vi "Remove Spurious.vi"(5 "Min V":dbl, 6 "Init":bool, 7 "Min I":dbl, 9 "VOLTS":dbl, 11 "Current":dbl) -> (0 "V Out":dbl, 3 "I Out":dbl)   [LabVIEW 2017]
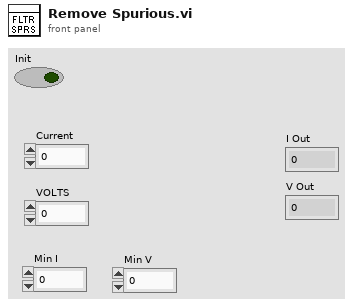
[diagram p1: front panel]
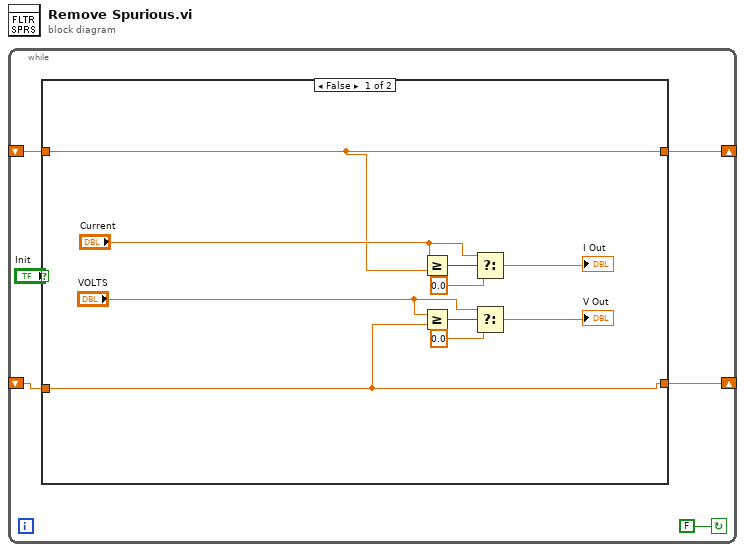
[diagram p0: block diagram]
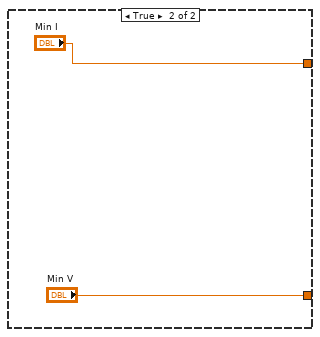
[diagram p2: hidden frame]
diagram:
  n1 = while {
    shift-right: [w3] -> _
    shift-left: _ -> [w2]
    shift-right: [w4] -> _
    shift-left: _ -> [w1]
    stop <- FALSE continue-if-true
    n2 = case shown="False" "Init" {
      tunnel: [w7 "Min V"] -> w4
      tunnel: [w8 "Min I"] -> w3
      tunnel: w2 -> [w8 _]
      tunnel: w1 -> [w7 _]
      frame False {
        n3 = Greater Or Equal?(x="Current", y=w8) -> (x >= y?=w11:bool)
        n4 = Greater Or Equal?(x="VOLTS", y=w7) -> (x >= y?=w15:bool)
        n5 = Select(t="Current", s=w11, f=0.0) -> (s? t:f=→"I Out":dbl)
        n6 = Select(t="VOLTS", s=w15, f=0.0) -> (s? t:f=→"V Out":dbl)
      }
      frame True {
      }
    }
  }
